vi "test_Add Command_Given Padding Lenght And Values Hidden When Pad is False.vi"(8 "error in (no error)":errorcluster, 11 "TestCase in":refnum<class "Instrument Addon Scripting API Messages Unit Tests.lvclass">) -> (0 "error out":errorcluster, 3 "TestCase out":refnum<class "Instrument Addon Scripting API Messages Unit Tests.lvclass">)   [LabVIEW 2018, in "Instrument Addon Scripting API Messages Unit Tests.lvclass"]
uses:
  Instrument Addon Scripting API Messages Unit Tests.lvclass
  Addon/Addon Shared/Types/Command Parameters.ctl
  Addon/Addon Shared/Types/Linked Channel Cluster.ctl
  Addon/Addon Shared/Types/FG Control.ctl
  APIs/Scripting API/TypeDefs/Command Settings.ctl
  <vilib>/NI Veristand/Custom Device API/Custom Device Item Ref.ctl
  APIs/Scripting API/TypeDefs/Padding.ctl
  NationalInstruments.VeriStand.SystemDefinitionAPI
  Addon/Addon Shared/SubVIs/Constants.vi
  <vilib>/NI/NI VeriStand Advanced SysDef API/_SubVIs/SysDef.Search.GUID.vi
  <vilib>/NI Veristand/Custom Device API/NI VeriStand - Get Item Property.vi
  <vilib>/NI Veristand/Custom Device API/Get Item Property (String).vi
  <vilib>/NI Veristand/Custom Device API/Get Item Property (String Array).vi
  <vilib>/NI Veristand/Custom Device API/Get Item Property (Boolean).vi
  <vilib>/NI Veristand/Custom Device API/Get Item Property (U32).vi
  <vilib>/NI Veristand/Custom Device API/NI VeriStand - Set Item Property.vi
  <vilib>/NI Veristand/Custom Device API/Set Item Property (String).vi
  <vilib>/NI Veristand/Custom Device API/Set Item Property (String Array).vi
  <vilib>/NI Veristand/Custom Device API/Set Item Property (Boolean).vi
  <vilib>/NI Veristand/Custom Device API/Set Item Property (U32).vi
  <vilib>/addons/_JKI Toolkits/VI Tester/TestCase.llb/TestCase.lvclass
  Instrument Addon Scripting API Test Assets/Instrument Addon Scripting API Test Assets.lvclass
  APIs/Scripting API/Instrument Addon Scripting API.lvlib
  Addon/Addon Shared/Instrument Addon Shared.lvlib
  <vilib>/NI/NI VeriStand Advanced SysDef API/SysDef API/Advanced System Definition.lvlib
  <vilib>/NI VeriStand/Custom Device API/Custom Device API.lvlib
  C:/Program Files (x86)/National Instruments/LabVIEW 2018/vi.lib/addons/_JKI Toolkits/VI Tester/TestCase.llb/TestCase.lvclass
panel:
  out "Command Parameters":T1={"Command"="", "Linked Channels"=[], "Pad"=FALSE, "Length"=25, "Pad Value"=0}
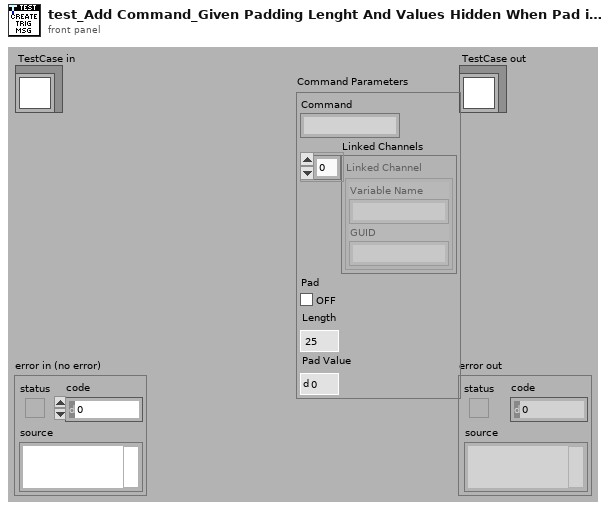
[diagram p1: front panel]
types:
  T1 = typedef "Instrument Addon Shared.lvlib/Command Parameters.ctl" = cluster{"Command":string, "Linked Channels":T2[], "Pad":bool, "Length":u32, "Pad Value":u8}
  T2 = typedef "Instrument Addon Shared.lvlib/Linked Channel Cluster.ctl" = cluster{"Variable Name":string, "GUID":string}
  T3 = typedef "Custom Device API.lvlib/Custom Device Item Ref.ctl" = u64
  T4 = cluster{"Variable Name":string, "Channel Ref in":T3}[]
  T5 = typedef "Instrument Addon Scripting API.lvlib/Command Settings.ctl" = cluster{"Command Format":string, "Linked Channels":cluster{"Variable Name":string, "Channel Ref in":T3}[], "Pad":bool, "Padding":T6}
  T6 = typedef "Instrument Addon Scripting API.lvlib/Padding.ctl" = cluster{"Pad Value":u8, "Length":u32}
  T7 = typedef "Instrument Addon Shared.lvlib/FG Control.ctl" = enum16{"Get", "Set"}
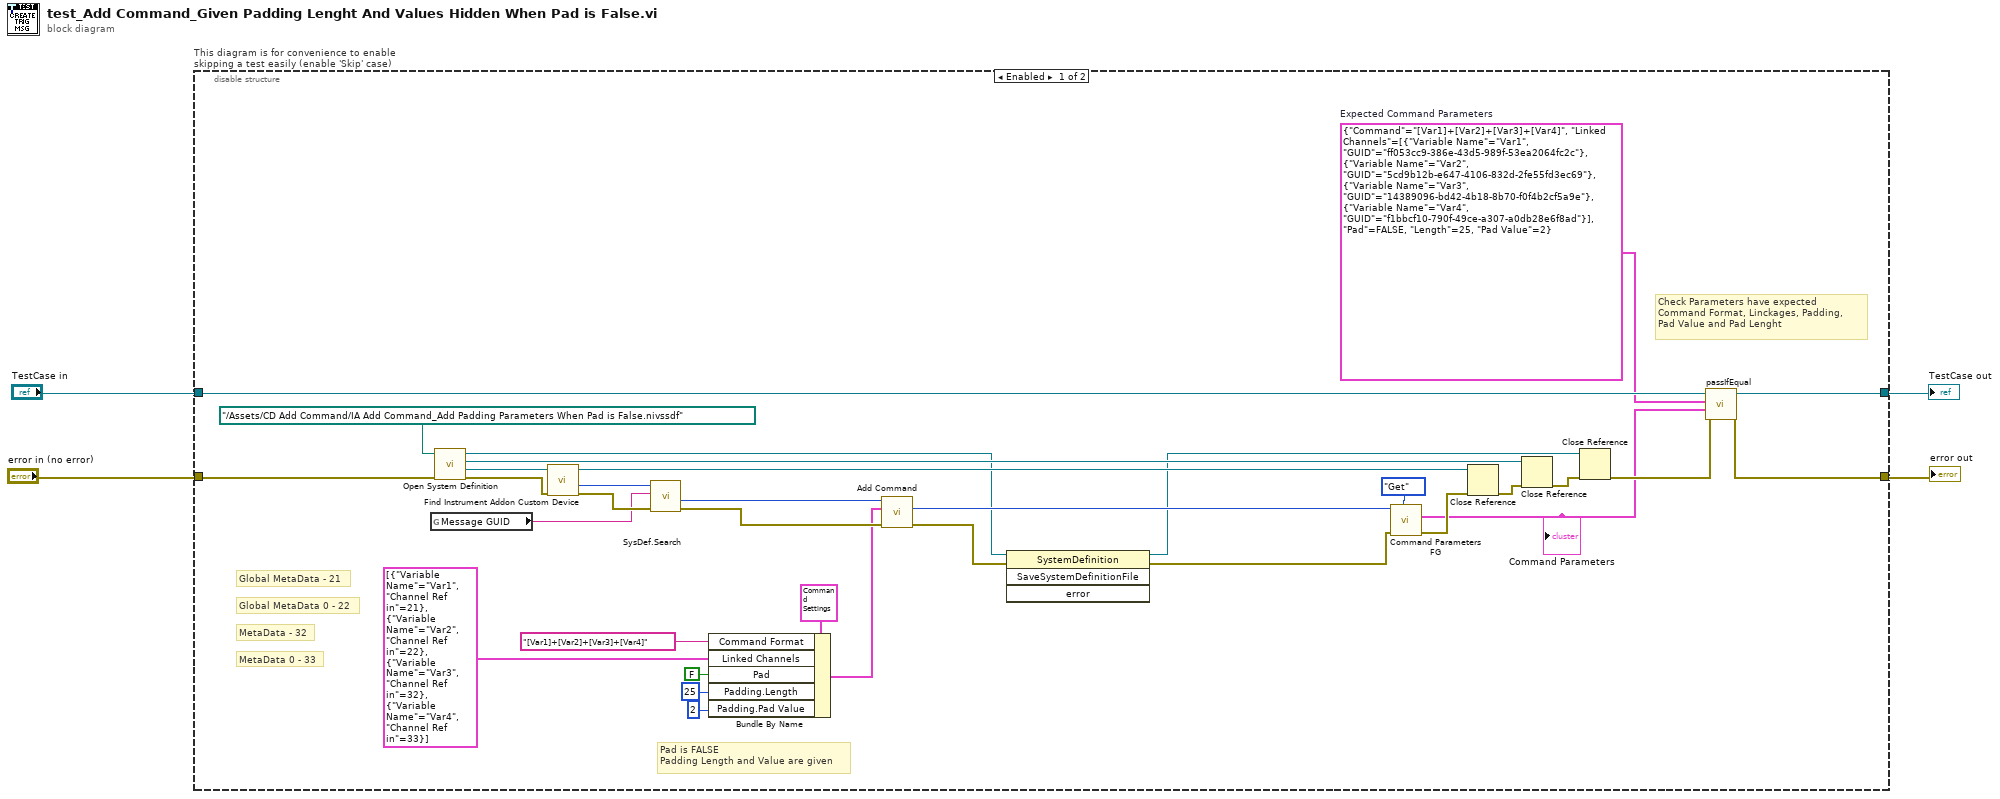
[diagram p0: block diagram]
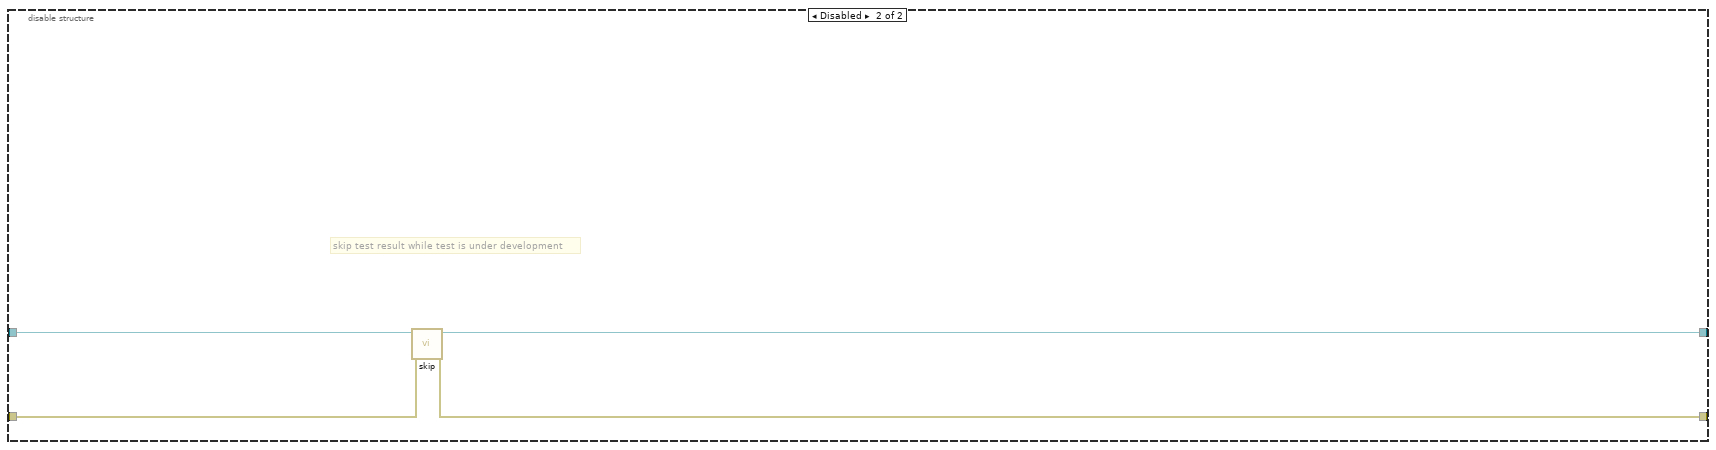
[diagram p2: hidden frame]
diagram:
  n1 = disable-structure "This diagram is for convenience to enable skipping a test easily (enable 'Skip' case)" shown="Enabled" {
    disable-tunnel: "TestCase in" -> [w34 w41]
    disable-tunnel: [w30 w39] -> w1
    disable-tunnel: [w31 w40] -> w3
    disable-tunnel: "error in (no error)" -> [w36 w38]
    frame Enabled {
      w13 = T1 {"Command"="[Var1]+[Var2]+[Var3]+[Var4]", "Linked Channels"=[{"Variable Name"="Var1", "GUID"="ff053cc9-386e-43d5-989f-53ea2064fc2c"}, {"Variable Name"="Var2", "GUID"="5cd9b12b-e647-4106-832d-2fe55fd3ec69"}, {"Variable Name"="Var3", "GUID"="14389096-bd42-4b18-8b70-f0f4b2cf5a9e"}, {"Variable Name"="Var4", "GUID"="f1bbcf10-790f-49ce-a307-a0db28e6f8ad"}], "Pad"=FALSE, "Length"=25, "Pad Value"=2}  # Expected Command Parameters
      # "Pad is FALSE\nPadding Length and Value are given"
      # "Check Parameters have expected \nCommand Format, Linckages, Padding,\nPad Value and Pad Lenght"
      # "MetaData 0 - 33"
      # "MetaData - 32"
      # "Global MetaData 0 - 22"
      # "Global MetaData - 21"
      n2 = global read "Constants.vi" "Message GUID"() -> (w21:string)
      n3 = call "Open System Definition.vi"("error in (no error)"=w36, "System Definition File"=path "../Assets/CD Add Command/IA Add Command_Add Padding Parameters When Pad is False.nivssdf" ("SDF file")) -> ("error out"=w23:errorcluster, "Target Refnum"=w24:refnum<k24>, "Root Refnum"=w35:refnum<k24>, "System Definition Refnum"=w8:refnum<k24>)  [unwired: 6 in]
      n4 = call "Find Instrument Addon Custom Device.vi"("error in"=w23, "target in"=w24) -> ("error out"=w22:errorcluster, "NodeID"=w14:u64, "target out"=w15:refnum<k24>)  [unwired: 7 in]
      n5 = call-poly <vilib>:"SysDef.Search.vi"("error in (no error)"=w22, "GUID"=w21, "nodeID"=w14) -> ("error out"=w20:errorcluster, "Value out"=w5:u64)  [unwired: 5 in, 2 out]
      n6 = Bundle By Name(cluster=T5 {"Command Format"="[Var1]+[Var2]", "Linked Channels"=[{"Variable Name"="Var1", "Channel Ref in"=32}, {"Variable Name"="Var2", "Channel Ref in"=33}], "Pad"=FALSE, "Padding"={"Pad Value"=0, "Length"=0}} ("Settings"), "Command Format"="[Var1]+[Var2]+[Var3]+[Var4]", "Linked Channels"=T4 [{"Variable Name"="Var1", "Channel Ref in"=21}, {"Variable Name"="Var2", "Channel Ref in"=22}, {"Variable Name"="Var3", "Channel Ref in"=32}, {"Variable Name"="Var4", "Channel Ref in"=33}], "Pad"=FALSE, "Padding.Length"=u32 25, "Padding.Pad Value"=u8 2) -> (w18:T5)
      n7 = call "Add Command.vi"("Error In"=w20, "Settings"=w18, "Message Refnum In"=w5) -> ("Error Out"=w9:errorcluster, "Command Refnum"=w27:T3)  [unwired: 6 in, 1 out]
      n8 = invoke class="SystemDefinition" method="SaveSystemDefinitionFile"(reference=w8, error in=w9) -> (reference out=w6:refnum<k24>, error out=w7:errorcluster)  [unwired: 2 in, 2 out]
      n9 = call "Command Parameters FG.vi"("Action"=FG_Control."Get", "error in (no error)"=w7, "Item Ref in"=w27) -> ("error out"=w26:errorcluster, "Command Parameters"=w25:T1)  [unwired: 6 in, 1 out]
      "Command Parameters" <- w25
      n10 = Close Reference(reference=w15, error in (no error)=w26) -> (error out=w29:errorcluster)
      n11 = Close Reference(reference=w35, error in (no error)=w29) -> (error out=w33:errorcluster)
      n12 = Close Reference(reference=w6, error in (no error)=w33) -> (error out=w32:errorcluster)
      n13 = call-dynamic "passIfEqual.vi"("error in (no error)"=w32, "y"=w25, "x"=w13, "TestCase in"=w34) -> ("error out"=w31:errorcluster, "TestCase out"=w30:refnum<class "Instrument Addon Scripting API Messages Unit Tests.lvclass">)  [unwired: 6 in]
    }
    frame Disabled {
      # "skip test result while test is under development"
      n14 = call <vilib>:"skip.vi"("error in (no error)"=w38, "TestCase in"=w41) -> ("error out"=w40:errorcluster, "TestCase out"=w39:refnum<class "Instrument Addon Scripting API Messages Unit Tests.lvclass">)  [unwired: 8 in]
    }
  }
  "error out" <- w3
  "TestCase out" <- w1
